vi "5_Recipe_u_1.vi"() -> ()   [LabVIEW 2011]
uses:
  Globals/Global VI.vi
  <vilib>/Utility/file.llb/Read From Spreadsheet File (string).vi
  <vilib>/Utility/file.llb/Write To Spreadsheet File (string).vi
  Globals/Global Recipe.vi
panel:
  out "recipe name":string
  out "Recipe in Use":string[][](table)
  in  "Use Recipe":bool
  out "save to path":path
  in  "Recipe Setup":string[][](table)
  in  "Save As Button":bool
  in  "Save Button":bool
  in  "Open Button":bool
  in  "New Button":bool
  # "Recipe"
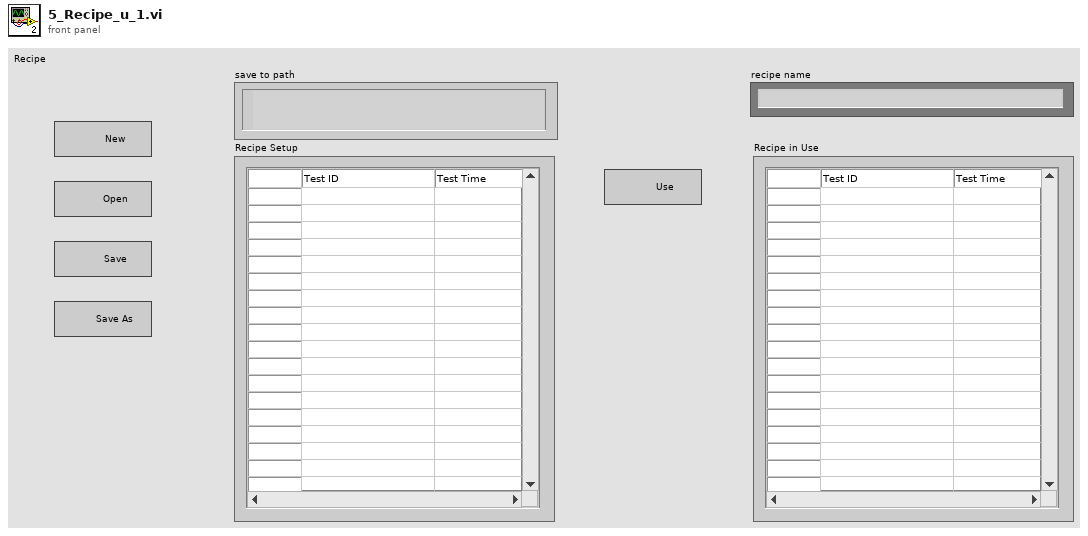
[diagram p1: front panel]
types:
  T1 = enum8{"Enabled", "Disabled", "Disabled and Grayed Out"}
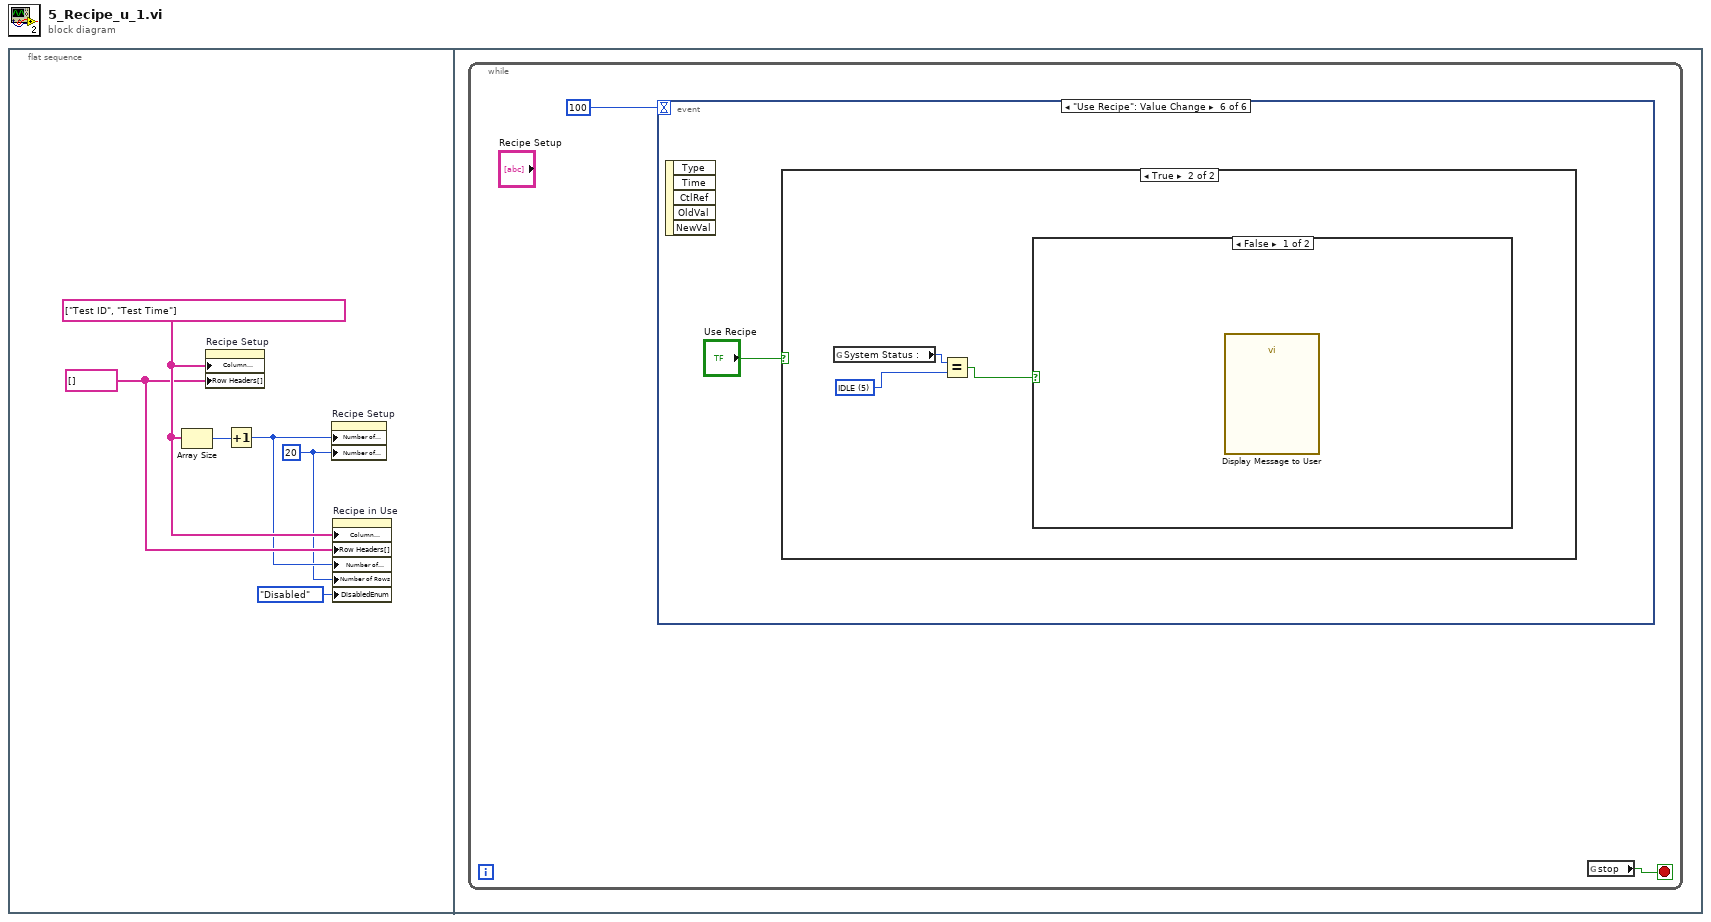
[diagram p0: block diagram]
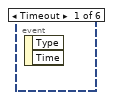
[diagram p2: hidden frame]
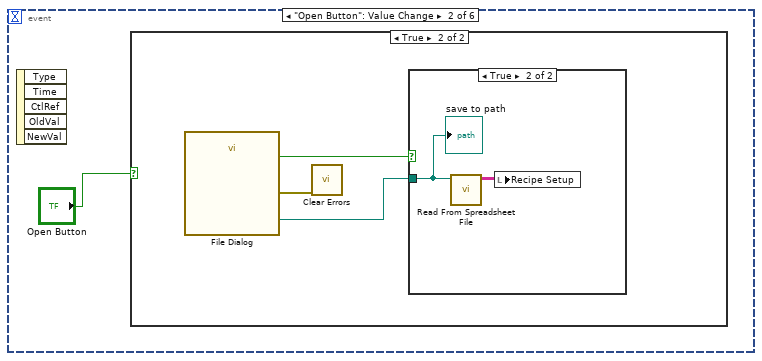
[diagram p3: hidden frame]
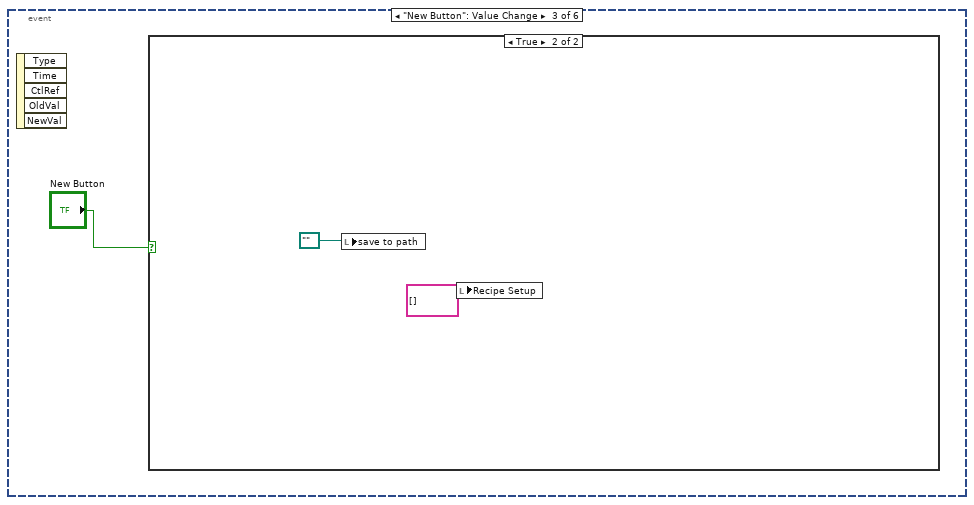
[diagram p6: hidden frame]
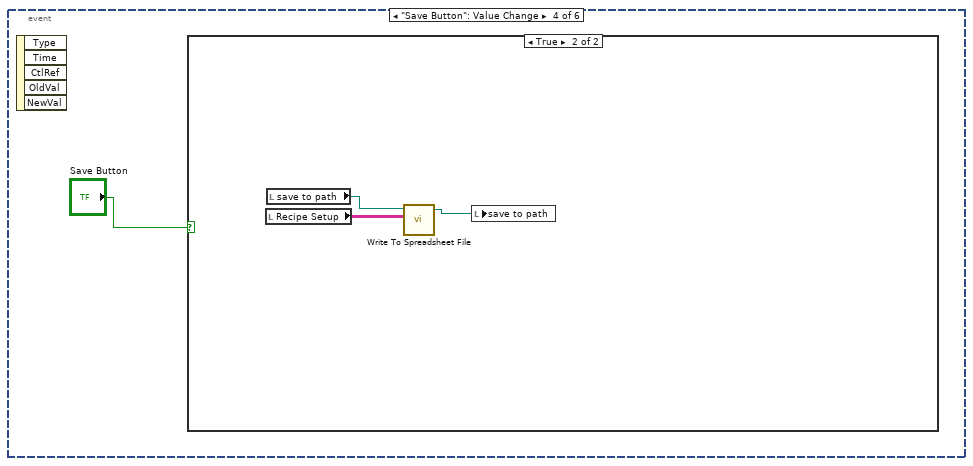
[diagram p8: hidden frame]
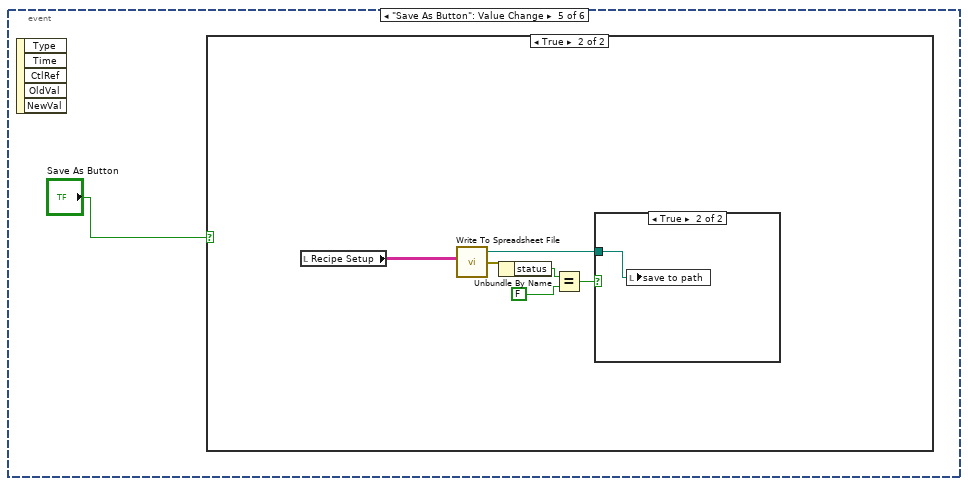
[diagram p10: hidden frame]
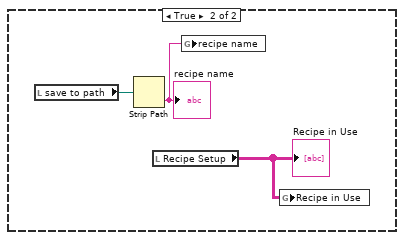
[diagram p14: hidden frame]
diagram:
  n1 = flat-sequence {
    frame #0 {
      w2 = u32 20 ("Number of Rows")
      w4 = string[] [] ("Row Header Strings[]")
      w5 = string[] ["Test ID", "Test Time"] ("Row Header Strings[]")
      n2 = Array Size(array=w5) -> (size(s)=w6:i32)
      n3 = property on="Recipe Setup" class="Tbl (strict)"("Column Headers[]"=w5, "Row Headers[]"=w4) -> ()  [unwired: 2 in, 2 out]
      n4 = Increment(x=w6) -> (x+1=w3:i32)
      n5 = property on="Recipe Setup" class="Tbl (strict)"("Number of Columns"=w3, "Number of Rows"=w2) -> ()  [unwired: 2 in, 2 out]
      n6 = property on="Recipe in Use" class="Tbl (strict)"("Column Headers[]"=w5, "Row Headers[]"=w4, "Number of Columns"=w3, "Number of Rows"=w2, "DisabledEnum"=T1."Disabled" ("Disabled")) -> ()  [unwired: 2 in, 2 out]
    }
    frame #1 {
      n7 = while {
        stop <- w8 stop-if-true
        n8 = event shown="[5] \"Use Recipe\": Value Change" {
          selector: _ -> [_ _ _ _ _ _]
          dyn-events: _ -> [_ _ _ _ _ _]
          timeout: 100 -> [_ _ _ _ _ _]
          event Timeout {
            n9 = event-data() -> ()  [unwired: 1 in, 2 out]
          }
          event "Open Button": Value Change {
            n10 = event-data() -> ()  [unwired: 1 in, 5 out]
            n11 = case shown="True" "Open Button" {
              frame False {
              }
              frame True {
                n12 = call "File Dialog"() -> ("selected path"=w12:path, "exists"=w11:bool, "error out"=w10:errorcluster)  [unwired: 12 in, 1 out]
                n13 = call <vilib>:"Clear Errors.vi"("error in (no error)"=w10) -> ()  [unwired: 6 in, 1 out]
                n14 = case shown="True" w11 {
                  tunnel: w12 -> [_ w14]
                  frame False {
                  }
                  frame True {
                    n15 = call-poly <vilib>:"Read From Spreadsheet File.vi"("file path (dialog if empty)"=w14) -> ("all rows"=w13:string[][])  [unwired: 6 in, 4 out]
                    n16 = local write "Recipe Setup"(w13) -> ()
                    "save to path" <- w14
                  }
                }
              }
            }
          }
          event "New Button": Value Change {
            n17 = event-data() -> ()  [unwired: 1 in, 5 out]
            n18 = case shown="True" "New Button" {
              frame False {
              }
              frame True {
                n19 = local write "save to path"(path "" ("selected path")) -> ()
                n20 = local write "Recipe Setup"(string[][] [] ("Item Names")) -> ()
              }
            }
          }
          event "Save Button": Value Change {
            n21 = event-data() -> ()  [unwired: 1 in, 5 out]
            n22 = case shown="True" "Save Button" {
              frame False {
              }
              frame True {
                n23 = local read "Recipe Setup"() -> (w21:string[][])
                n24 = local read "save to path"() -> (w20:path)
                n25 = call-poly <vilib>:"Write To Spreadsheet File.vi"("2D data"=w21, "file path (dialog if empty)"=w20) -> ("new file path (Not A Path if cancelled)"=w19:path)  [unwired: 5 in, 1 out]
                n26 = local write "save to path"(w19) -> ()
              }
            }
          }
          event "Save As Button": Value Change {
            n27 = event-data() -> ()  [unwired: 1 in, 5 out]
            n28 = case shown="True" "Save As Button" {
              frame False {
              }
              frame True {
                n29 = local read "Recipe Setup"() -> (w28:string[][])
                n30 = call-poly <vilib>:"Write To Spreadsheet File.vi"("2D data"=w28) -> ("error out"=w26:errorcluster, "new file path (Not A Path if cancelled)"=w27:path)  [unwired: 6 in]
                n31 = Unbundle By Name(w26) -> ("status"=w25:bool)
                n32 = Equal?(x=w25, y=FALSE ("status")) -> (x = y?=w23:bool)
                n33 = case shown="True" w23 {
                  tunnel: w27 -> [_ w29]
                  frame False {
                  }
                  frame True {
                    n34 = local write "save to path"(w29) -> ()
                  }
                }
              }
            }
          }
          event "Use Recipe": Value Change {
            n35 = event-data() -> ()  [unwired: 1 in, 5 out]
            n36 = case shown="True" "Use Recipe" {
              frame False {
              }
              frame True {
                w33 = u16 5 items=["NOT READY", "E-STOPPED", "FAULTED", "PAUSING...", "PAUSED", "IDLE", "RUNNING", "UNCALIBRATED", "CALIBRATING...", "POWER OFF", "POWERING ON...", "MANUAL MODE", "CONNECTING..."] ("System Status :")
                n37 = global read "Global Recipe.vi" "System Status :"() -> (w32:u16)
                n38 = Equal?(x=w32, y=w33) -> (x = y?=w31:bool)
                n39 = case shown="False" w31 {
                  frame False {
                    n40 = call "Display Message to User"() -> ()  [unwired: 10 in, 2 out]
                  }
                  frame True {
                    n41 = local read "save to path"() -> (w36:path)
                    n42 = Strip Path(path=w36) -> (name=w35:string)  [unwired: 1 out]
                    "recipe name" <- w35
                    n43 = local read "Recipe Setup"() -> (w34:string[][])
                    "Recipe in Use" <- w34
                    n44 = global write "Global Recipe.vi" "recipe name"(w35) -> ()
                    n45 = global write "Global Recipe.vi" "Recipe in Use"(w34) -> ()
                  }
                }
              }
            }
          }
        }
        n46 = global read "Global VI.vi" "stop"() -> (w8:bool)
      }
    }
  }
